vi "DatabaseWrite SubVI.vi"(0 "Input name of the new user":string, 2 "String":string, 5 "Input second name of the new user":string, 7 "Input":string, 9 "Image path to the users biometrics":string, 11 "error in (no error)":errorcluster) -> (15 "error out":errorcluster)   [LabVIEW 2024]
doc: "SubVi odpowiedzialne za wpisywanie wartości do bazy danych"
uses:
  <vilib>/addons/database/Connection.llb/DB Tools Open Connec (Path).vi
  <vilib>/addons/database/NI_Database_API.lvlib
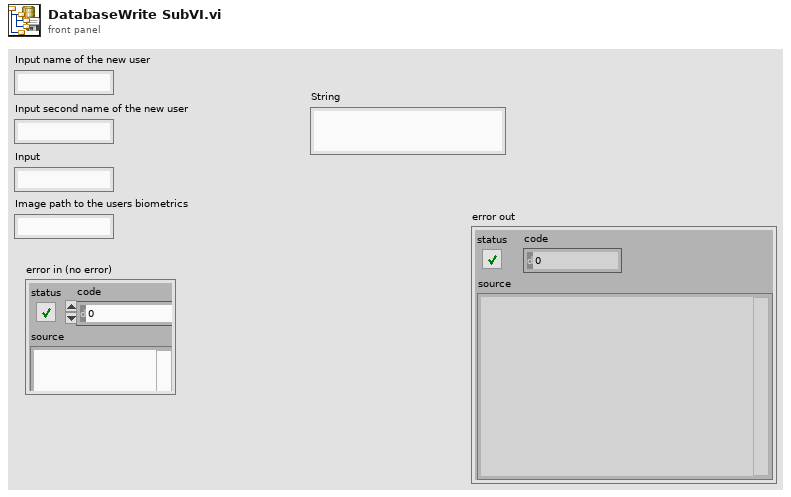
[diagram p1: front panel]
types:
  T1 = typedef "NI_Database_API.lvlib/Conn ObjectReference.ctl" = refnum<k1>
  T2 = cluster{"Input name of the new user":string, "Input second name of the new user":string, "Input":string, "Image path to the users biometrics":string}
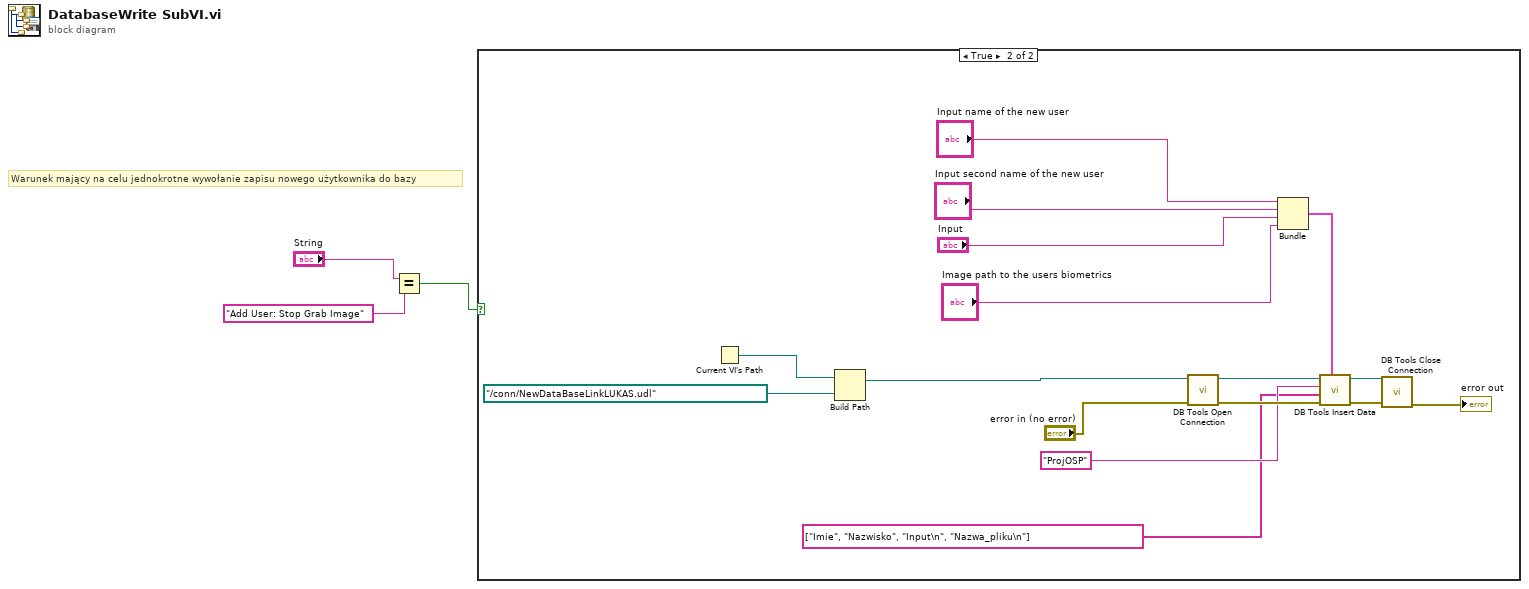
[diagram p0: block diagram]
diagram:
  # "Warunek mający na celu jednokrotne wywołanie zapisu nowego użytkownika do bazy"
  n1 = Equal?(x="String", y="Add User: Stop Grab Image") -> (x = y?=w1:bool)
  n2 = case shown="True" w1 {
    frame False {
    }
    frame True {
      n3 = Current VI's Path() -> (path=w11:path)
      n4 = Build Path(base path=w11, name or relative path=path "../conn/NewDataBaseLinkLUKAS.udl") -> (appended path=w9:path)
      n5 = call-poly <vilib>:"DB Tools Open Connection.vi"("error in (no error)"="error in (no error)", "connection information"=w9) -> ("error out"=w19:errorcluster, "connection reference"=w17:T1)  [unwired: 6 in]
      n6 = Bundle("Input name of the new user"="Input name of the new user", "Input second name of the new user"="Input second name of the new user", "Input"="Input", "Image path to the users biometrics"="Image path to the users biometrics") -> (w14:T2)  [unwired: 1 in]
      n7 = call <vilib>:"DB Tools Insert Data.vi"("data"=w14, "error in (no error)"=w19, "columns"=string[] ["Imie", "Nazwisko", "Input\n", "Nazwa_pliku\n"], "table"="ProjOSP", "connection reference"=w17) -> ("error out"=w18:errorcluster, "connection reference out"=w16:T1)  [unwired: 5 in]
      n8 = call <vilib>:"DB Tools Close Connection.vi"("error in (no error)"=w18, "connection reference"=w16) -> ("error out"=→"error out":errorcluster)  [unwired: 5 in]
    }
  }
